vi "recondense_Queue_Commands.vi"(1 "Recondense-Control":T1, 3 "16T Queue":refnum<queue>) -> (0 "Recondense-Control new status":T1)   [LabVIEW 2019]
uses:
  Brosowski/Borowski-Control-Cluster.ctl
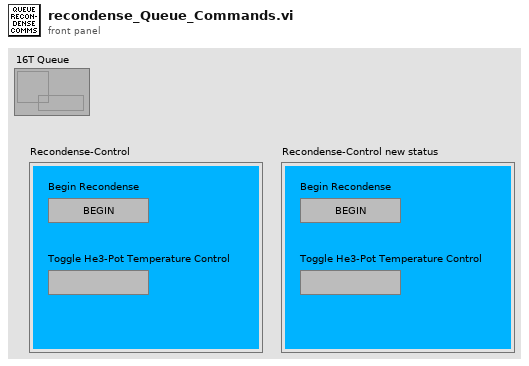
[diagram p1: front panel]
types:
  T1 = typedef "Borowski-Control-Cluster.ctl" = cluster{"Begin Recondense":bool, "Toggle He3-Pot Temperature Control":bool}
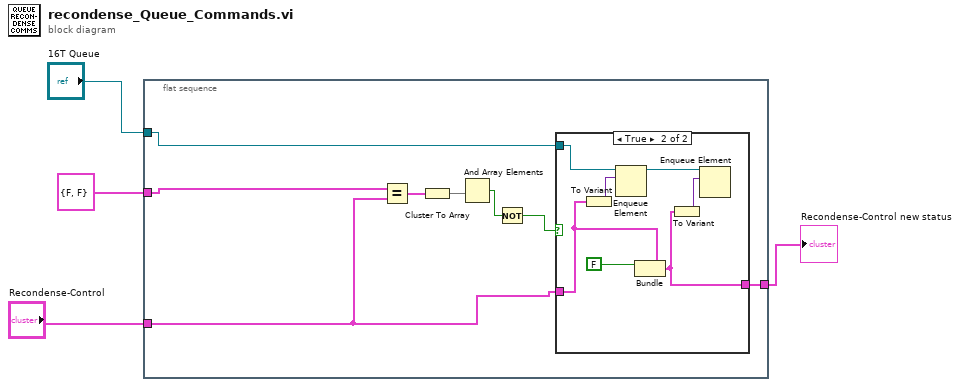
[diagram p0: block diagram]
diagram:
  n1 = flat-sequence {
    tunnel: "16T Queue" -> [w12]
    tunnel: T1 {"Begin Recondense"=FALSE, "Toggle He3-Pot Temperature Control"=FALSE} ("Recondense-Control") -> [w11]
    tunnel: "Recondense-Control" -> [w5]
    tunnel: [w6] -> w1
    frame #0 {
      n2 = Equal?(x=w11, y=w5) -> (x = y?=w10:T1)
      n3 = Cluster To Array(cluster=w10) -> (array=w9:bool[])
      n4 = And Array Elements(Boolean array=w9) -> (logical AND=w8:bool)
      n5 = Not(x=w8) -> (.not. x?=w7:bool)
      n6 = case shown="True" w7 {
        tunnel: w12 -> [_ w20]
        tunnel: w5 -> [w13 w18]
        tunnel: [w13 w17] -> w6
        frame False {
        }
        frame True {
          n7 = To Variant(anything=w18) -> (Variant=w19:variant)
          n8 = Enqueue Element(queue=w20, element=w19) -> (queue out=w15:refnum<queue>)  [unwired: 2 in, 2 out]
          n9 = Bundle(cluster=w18, "Begin Recondense"=FALSE) -> (w17:T1)  [unwired: 1 in]
          n10 = To Variant(anything=w17) -> (Variant=w16:variant)
          n11 = Enqueue Element(queue=w15, element=w16) -> ()  [unwired: 2 in, 3 out]
        }
      }
    }
  }
  "Recondense-Control new status" <- w1
